vi "NI VeriStand - Open Macro Recorder Reference.vi"(8 "error in (no error)":errorcluster) -> (0 "error out":errorcluster, 3 "MacroRecorder":T1)   [LabVIEW 2020, in "NI_VS MacroRecorderAPI.lvlib"]
doc: "Opens a reference to the Macro Recorder tool on the VeriStand Gateway. You must open a reference before using any other VIs on this palette."
uses:
  <vilib>/NI VeriStand/Execution/MacroRecorder/NI_VS MacroRecorderAPI.lvlib
  <vilib>/NI VeriStand/Execution/MacroRecorder/MacroRecorderAPI.ctl
  NationalInstruments.VeriStand.ClientAPI
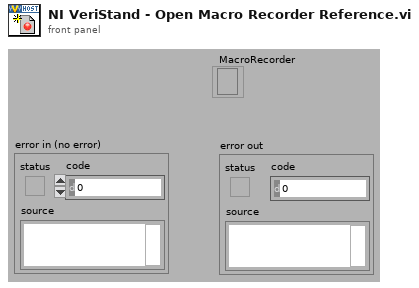
[diagram p1: front panel]
types:
  T1 = typedef "NI_VS MacroRecorderAPI.lvlib/MacroRecorderAPI.ctl" = refnum<k24>
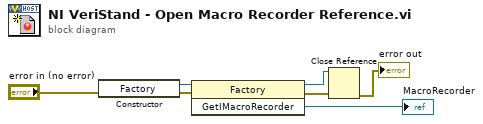
[diagram p0: block diagram]
diagram:
  n1 = constructor class="Factory"(error in="error in (no error)") -> (reference out=w6:refnum<k24>, error out=w7:errorcluster)  [unwired: 2 in, 1 out]
  n2 = invoke class="Factory" method="GetIMacroRecorder"(reference=w6, error in=w7) -> (reference out=w4:refnum<k24>, error out=w5:errorcluster, "GetIMacroRecorder"=→"MacroRecorder":refnum<k24>)  [unwired: 1 in]
  n3 = Close Reference(reference=w4, error in (no error)=w5) -> (error out=→"error out":errorcluster)
